vi "Mod5.vi"() -> ()   [LabVIEW 2014]
uses:
  <vilib>/myRIO/Instrument Drivers/Onboard IO/DIO/vis/Read.vi
  <vilib>/myRIO/Common/Instrument Driver Framework/myRIO v1.0/UART/vis/myRIO v1.0 Close UART.vi
  <vilib>/myRIO/Instrument Drivers/Onboard IO/DIO/vis/Smart Open.vi
  <vilib>/Utility/error.llb/Error Cluster From Error Code.vi
  <vilib>/myRIO/Common/Instrument Driver Framework/myRIO v1.0/DIO/vis/myRIO v1.0 Read DIO.vi
  <vilib>/myRIO/Common/Instrument Driver Framework/Utilities/vis/FPGA Ref Manager.vi
  <vilib>/myRIO/Common/Instrument Driver Framework/myRIO v1.0/myRIO v1.0 Reset FPGA.vi
  <vilib>/myRIO/Common/Instrument Driver Framework/myRIO v1.0/IRQ/vis/myRIO v1.0 IRQ Info FGV.vi
  <vilib>/myRIO/Common/Instrument Driver Framework/myRIO v1.0/IRQ/vis/myRIO v1.0 Timer IRQ Info FGV.vi
  <vilib>/myRIO/Common/Instrument Driver Framework/myRIO v1.0/IRQ/vis/myRIO v1.0 ISR Agent.vi
  <vilib>/myRIO/Instrument Drivers/Utilities/Utilities.lvlib
panel:
  out "B/DIO0 presses/releases":i32
  out "C/DIO0 state":bool
  out "B/DIO0 state":bool
  out "A/DIO0 state":bool
  # "Pushbutton demo"
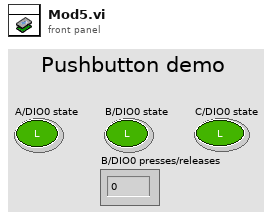
[diagram p1: front panel]
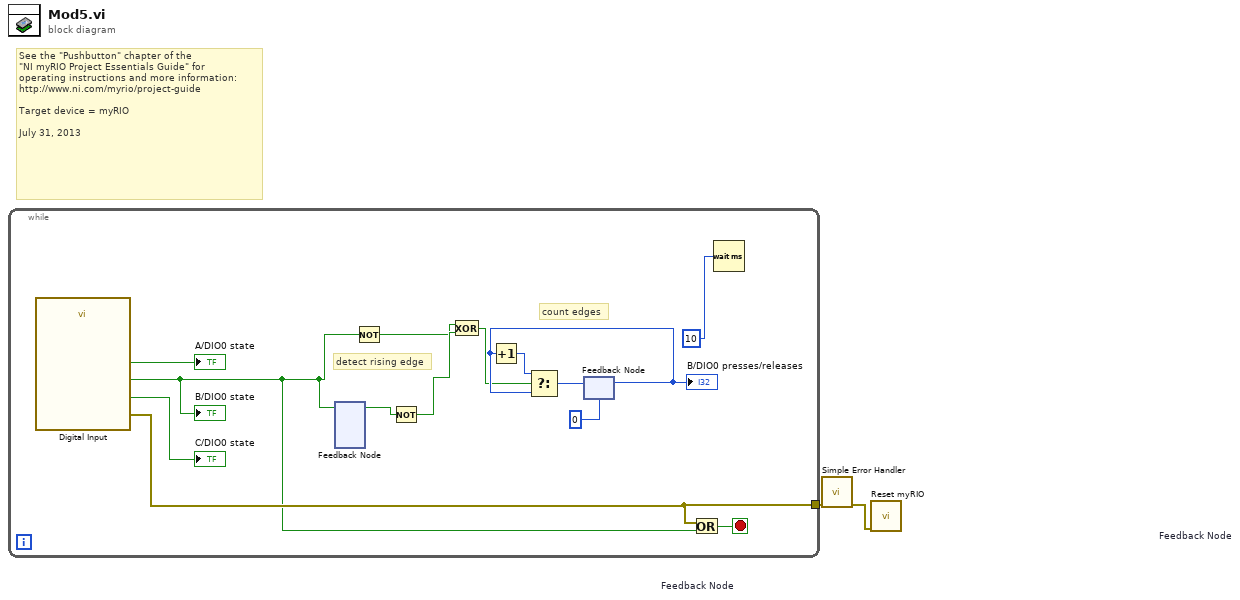
[diagram p0: block diagram]
diagram:
  # "See the \"Pushbutton\" chapter of the\n\"NI myRIO Project Essentials Guide\" for\noperating instructions and more information: \nhttp://www.ni.com/myrio/project-guide\n\nTarget device = myRIO\n\nJuly 31, 2013"
  n1 = while {
    tunnel: [w14] -> w2
    stop <- w16 stop-if-true
    # "count edges"
    # "detect rising edge"
    n2 = call "Digital Input"() -> ("A/DIO0 (Pin 11)"=→"A/DIO0 state":bool, "B/DIO0 (Pin 11)"=w3:bool, "C/DIO0"=→"C/DIO0 state":bool, "error out"=w14:errorcluster)  [unwired: 24 in]
    "B/DIO0 state" <- w3
    n3 = feedback-in #1(w3) -> ()
    n4 = feedback #1 "Feedback Node"() -> (w7:bool)  [unwired: 1 in]
    n5 = Not(x=w3) -> (.not. x?=w4:bool)
    n6 = Not(x=w7) -> (.not. x?=w5:bool)
    n7 = Exclusive Or(1:w5, 2:w4) -> (0:w6:bool)
    n8 = feedback #2 "Feedback Node"(0) -> (w8:i32)
    "B/DIO0 presses/releases" <- w8
    n9 = Increment(x=w8) -> (x+1=w10:i32)
    n10 = Select(t=w10, s=w6, f=w8) -> (s? t:f=w9:i32)
    n11 = feedback-in #2(w9) -> ()
    n12 = Or(x=w14, y=w3) -> (x .or. y?=w16:bool)
    n13 = Wait (ms)(milliseconds to wait=u32 10) -> ()  [unwired: 1 out]
  }
  n14 = call <vilib>:"Simple Error Handler.vi"("error in (no error)"=w2) -> ("error out"=w1:errorcluster)  [unwired: 4 in, 4 out]
  n15 = call <vilib>:"Reset myRIO.vi"("error in (no error)"=w1) -> ()  [unwired: 10 in, 1 out]
